vi "ELVIS III v1.1 Start AO Continuous.vi"(8 "error in (no error)":errorcluster, 9 "AO FIFO Sample Rate":dbl=1000.0 min=1000.0 max=1600000.0, 10 "Channel Info":T1, 11 "myRIO Ref In":T2) -> (0 "error out":errorcluster, 2 "Channel Info Out":T1, 3 "myRIO Ref Out":T2)   [LabVIEW 2021]
uses:
  <vilib>/myRIO/Common/Instrument Driver Framework/Utilities/typedefs/myRIO v1.0 Reference.ctl
  <vilib>/myRIO/Common/Instrument Driver Framework/Utilities/typedefs/Generic FPGA Reference.ctl
  <vilib>/myRIO/Common/Instrument Driver Framework/ELVIS III v1.0/AO Continuous/typedefs/AO Continuous Channel Info.ctl
  <vilib>/myRIO/Common/Instrument Driver Framework/ELVIS III v1.0/AO Block/typedefs/ELVIS III AO Block Channels FPGA Reference.ctl
  <vilib>/rvi/errors/niLvFpgaAdjustHostInterfaceError.vi
  <vilib>/rvi/interface/nirviReadWriteControl/nirviReadWriteControl.xnode
  NiFpgaLv.dll
  <vilib>/rvi/interface/Simulation/niFpgaSimulationCallBeginRW.vi
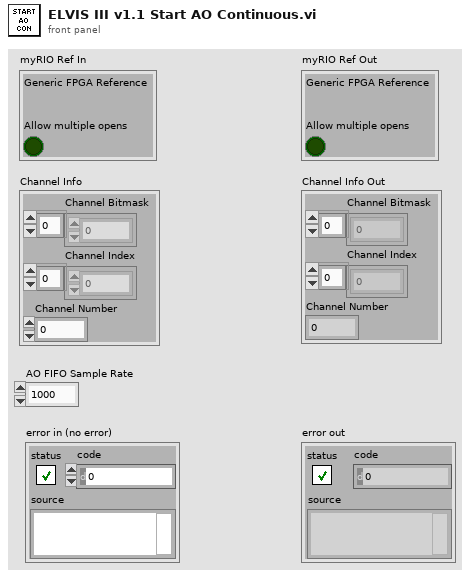
[diagram p1: front panel]
types:
  T1 = typedef "AO Continuous Channel Info.ctl" = cluster{"Channel Bitmask":u8[], "Channel Index":i32[], "Channel Number":u8}
  T2 = typedef "myRIO v1.0 Reference.ctl" = cluster{"Generic FPGA Reference":T3, "Allow multiple opens":bool}
  T3 = typedef "Generic FPGA Reference.ctl" = refnum<k20>
  T4 = typedef "ELVIS III AO Block Channels FPGA Reference.ctl" = refnum<k20>
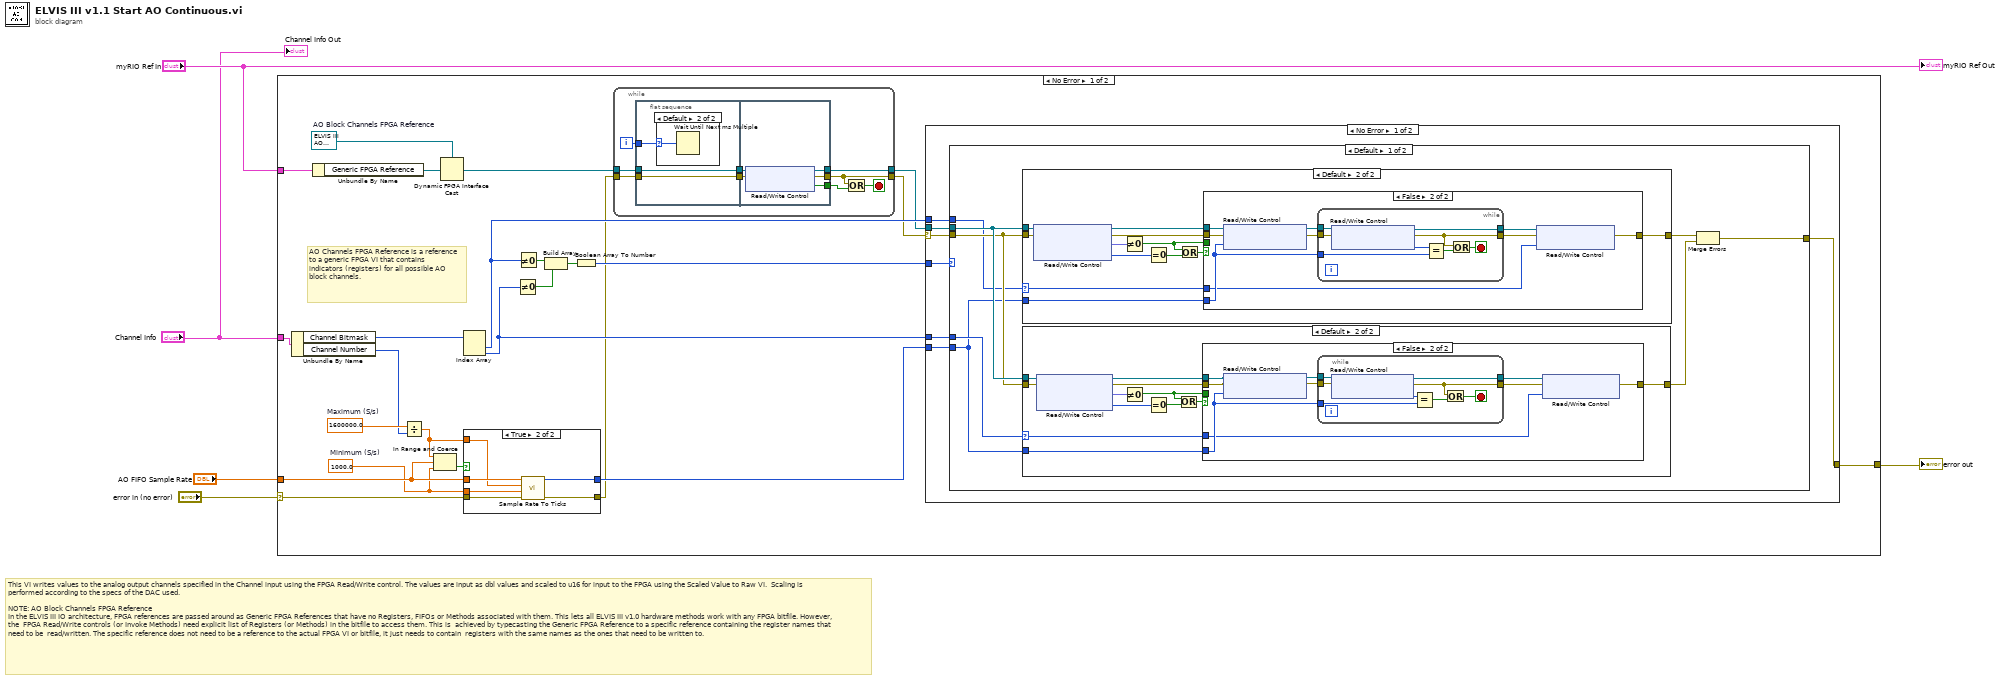
[diagram p0: block diagram]
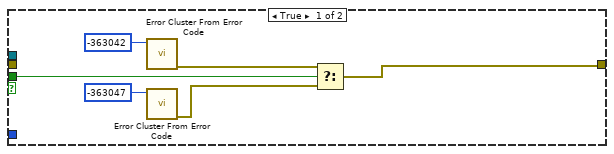
[diagram p3: hidden frame]
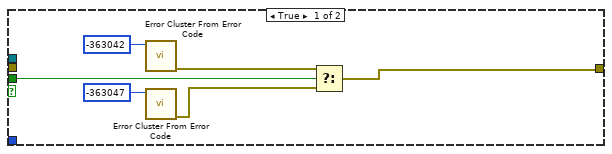
[diagram p5: hidden frame]
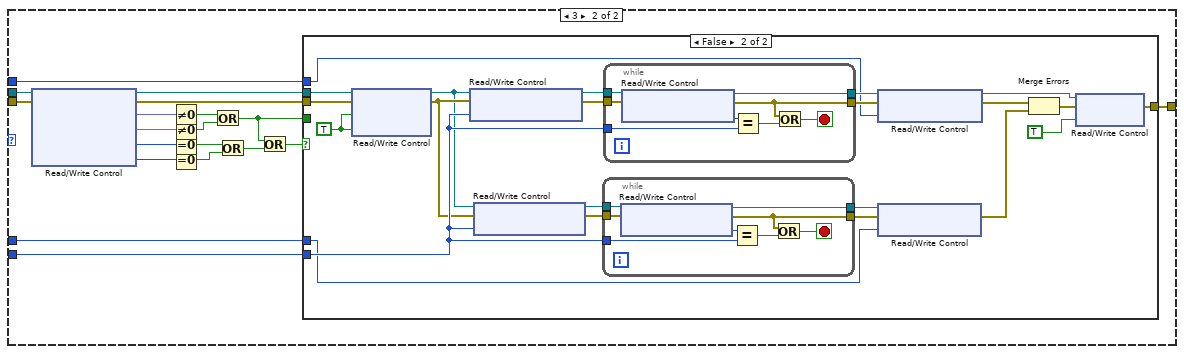
[diagram p6: hidden frame]
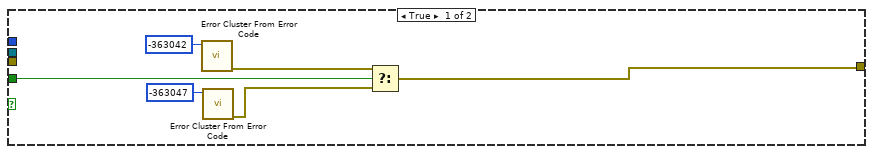
[diagram p7: hidden frame]
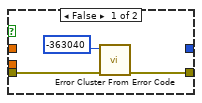
[diagram p10: hidden frame]
diagram:
  # "This VI writes values to the analog output channels specified in the Channel input using the FPGA Read/Write control. The values are input as dbl values and scaled to u16 for input to the FPGA using the Scaled Value to Raw VI.  Scaling is performed according to the specs of the DAC used.\n\nNOTE: AO Block Channels FPGA Reference\nIn the ELVIS III IO architecture, FPGA references are passed around as Generic FPGA References that have no Registers, FIFOs or Methods associated with them. This lets all ELVIS III v1.0 hardware methods work with any FPGA bitfile. However, the  FPGA Read/Write controls (or Invoke Methods) need explicit list of Registers (or Methods) in the bitfile to access them. This is  achieved by typecasting the Generic FPGA Reference to a specific reference containing the register names that need to be  read/written. The specific reference does not need to be a reference to the actual FPGA VI or bitfile, it just needs to contain  registers with the same names as the ones that need to be written to."
  n1 = case shown="No Error" "error in (no error)" {
    selector: "error in (no error)" -> [w13 w208]
    tunnel: [w14 w208] -> w5
    tunnel: "AO FIFO Sample Rate" -> [w26 _]
    tunnel: "myRIO Ref In" -> [w28 _]
    tunnel: "Channel Info" -> [w18 _]
    frame No Error {
      w24 = 1000.0  # Minimum (S/s)
      w12 = 1600000.0  # Maximum (S/s)
      w27 = T4 refnum  # AO Block Channels FPGA Reference
      # "AO Channels FPGA Reference is a reference to a generic FPGA VI that contains indicators (registers) for all possible AO block channels."
      n2 = Unbundle By Name(w18) -> ("Channel Bitmask"=w17:u8[], "Channel Number"=w11:u8)
      n3 = Unbundle By Name(w28) -> ("Generic FPGA Reference"=w29:T3)
      n4 = Divide(x=w12, y=w11) -> (x/y=w10:dbl)
      n5 = In Range and Coerce(upper limit=w10, x=w26, lower limit=w24) -> (In Range?=w25:bool)  [unwired: 1 out]
      n6 = Dynamic FPGA Interface Cast(Session In=w27, Type=w29) -> (Session Out=w9:T4)
      n7 = Index Array(array=w17) -> (element #1=w16:u8, element #2=w15:u8)  [unwired: 2 in]
      n8 = case shown="True" w25 {
        tunnel: [_ w207] -> w19
        tunnel: w13 -> [w200 w206]
        tunnel: [w199 w205] -> w8
        tunnel: w26 -> [_ w204]
        tunnel: w24 -> [_ w203]
        tunnel: w10 -> [_ w202]
        frame False {
          n9 = call <vilib>:"Error Cluster From Error Code.vi"("error in (no error)"=w200, "error code (0)"=-363040) -> ("error out"=w199:errorcluster)  [unwired: 7 in]
        }
        frame True {
          n10 = call <vilib>:"Sample Rate To Ticks.vi"("error in (no error)"=w206, "Minimum (S/s)"=w203, "Maximum (S/s)"=w202, "Sample Rate (S/s)"=w204) -> ("error out"=w205:errorcluster, "Count (tick/s)"=w207:u32)  [unwired: 5 in, 1 out]
        }
      }
      n11 = Not Equal To 0?(x=w15) -> (x != 0?=w21:bool)
      n12 = Not Equal To 0?(x=w16) -> (x != 0?=w22:bool)
      n13 = Build Array(w22, w21) -> (w23:bool[])
      n14 = Boolean Array To Number(Boolean array=w23) -> (number=w20:u32)
      n15 = while {
        tunnel: w9 -> [w189]
        tunnel: w8 -> [w188]
        tunnel: [w184] -> w6
        tunnel: [w187] -> w7
        i -> [w181]
        stop <- w182 stop-if-true
        n16 = flat-sequence {
          tunnel: w188 -> [w191]
          tunnel: w189 -> [w192]
          tunnel: [w192] -> w186
          tunnel: [w191] -> w185
          tunnel: w181 -> [w190]
          tunnel: [w196] -> w183
          tunnel: [w195] -> w184
          tunnel: [w194] -> w187
          tunnel: w186 -> [w198]
          tunnel: w185 -> [w197]
          frame #0 {
            n17 = case shown="Default" w190 {
              selector: w190 -> [_ w193]
              frame 0 {
              }
              frame Default {
                n18 = Wait Until Next ms Multiple(millisecond multiple=w193) -> ()  [unwired: 1 out]
              }
            }
          }
          frame #1 {
            n19 = xnode "Read/Write Control"("FPGA VI Reference In"=w198, "error in"=w197) -> ("FPGA VI Reference Out"=w194:T4, "error out"=w195:errorcluster, "DMA.SYS.RDY"=w196:bool)
          }
        }
        n20 = Or(x=w184, y=w183) -> (x .or. y?=w182:bool)
      }
      n21 = case shown="No Error" w6 {
        selector: w6 -> [w30 w180]
        tunnel: w20 -> [w36 _]
        tunnel: w19 -> [w35 _]
        tunnel: w16 -> [w34 _]
        tunnel: w15 -> [w33 _]
        tunnel: [w32 w180] -> w14
        tunnel: w7 -> [w31 _]
        frame No Error {
          n22 = case shown="Default" w36 {
            tunnel: w31 -> [w44 w129]
            tunnel: w30 -> [w43 w128]
            tunnel: w34 -> [w42 w132]
            tunnel: w35 -> [w40 w135]
            tunnel: w33 -> [w41 w134]
            tunnel: [w39 w133] -> w32
            frame Default {
              n23 = case shown="Default" w42 {
                selector: w42 -> [_ w93]
                tunnel: w44 -> [_ w90]
                tunnel: w43 -> [w81 w89]
                tunnel: w40 -> [_ w92]
                tunnel: [w81 w91] -> w38
                frame 0 {
                }
                frame Default {
                  n24 = xnode "Read/Write Control"("FPGA VI Reference In"=w90, "error in"=w89) -> ("FPGA VI Reference Out"=w87:T4, "error out"=w88:errorcluster, "AO.A.DMA_ENA"=w86:fxp<+,2,2>, "AO.A.ELE_NUM"=w83:u32)
                  n25 = Not Equal To 0?(x=w86) -> (x != 0?=w84:bool)
                  n26 = Equal To 0?(x=w83) -> (x = 0?=w82:bool)
                  n27 = Or(x=w84, y=w82) -> (x .or. y?=w85:bool)
                  n28 = case shown="False" w85 {
                    tunnel: w88 -> [_ w107]
                    tunnel: [w96 w101] -> w91
                    tunnel: w87 -> [_ w108]
                    tunnel: w93 -> [_ w100]
                    tunnel: w92 -> [_ w104]
                    tunnel: w84 -> [w98 _]
                    frame True {
                      n29 = call <vilib>:"Error Cluster From Error Code.vi"("error code (0)"=-363042) -> ("error out"=w97:errorcluster)  [unwired: 8 in]
                      n30 = call <vilib>:"Error Cluster From Error Code.vi"("error code (0)"=-363047) -> ("error out"=w94:errorcluster)  [unwired: 8 in]
                      n31 = Select(t=w97, s=w98, f=w94) -> (s? t:f=w96:errorcluster)
                    }
                    frame False {
                      n32 = xnode "Read/Write Control"("FPGA VI Reference In"=w108, "error in"=w107, "AO.A.DMA_CNTR"=w104) -> ("FPGA VI Reference Out"=w106:T4, "error out"=w105:errorcluster)
                      n33 = while {
                        tunnel: w106 -> [w116]
                        tunnel: [w115] -> w103
                        tunnel: [w111] -> w102
                        tunnel: w105 -> [w114]
                        tunnel: w104 -> [w112]
                        stop <- w110 stop-if-true
                        n34 = xnode "Read/Write Control"("FPGA VI Reference In"=w116, "error in"=w114) -> ("FPGA VI Reference Out"=w115:T4, "error out"=w111:errorcluster, "AO.A.DMA_CNTR"=w113:u32)
                        n35 = Equal?(x=w113, y=w112) -> (x = y?=w109:bool)
                        n36 = Or(x=w111, y=w109) -> (x .or. y?=w110:bool)
                      }
                      n37 = xnode "Read/Write Control"("FPGA VI Reference In"=w103, "error in"=w102, "AO.A.DMA_ENA"=w100) -> ("error out"=w101:errorcluster)  [unwired: 1 out]
                    }
                  }
                }
              }
              n38 = case shown="Default" w41 {
                selector: w41 -> [_ w57]
                tunnel: w44 -> [_ w54]
                tunnel: w43 -> [w45 w53]
                tunnel: w40 -> [_ w56]
                tunnel: [w45 w55] -> w37
                frame 0 {
                }
                frame Default {
                  n39 = xnode "Read/Write Control"("FPGA VI Reference In"=w54, "error in"=w53) -> ("FPGA VI Reference Out"=w51:T4, "error out"=w50:errorcluster, "AO.B.DMA_ENA"=w52:fxp<+,2,2>, "AO.B.ELE_NUM"=w47:u32)
                  n40 = Not Equal To 0?(x=w52) -> (x != 0?=w48:bool)
                  n41 = Equal To 0?(x=w47) -> (x = 0?=w46:bool)
                  n42 = Or(x=w48, y=w46) -> (x .or. y?=w49:bool)
                  n43 = case shown="False" w49 {
                    tunnel: w50 -> [_ w71]
                    tunnel: [w58 w64] -> w55
                    tunnel: w51 -> [_ w72]
                    tunnel: w57 -> [_ w67]
                    tunnel: w56 -> [_ w68]
                    tunnel: w48 -> [w62 _]
                    frame True {
                      n44 = call <vilib>:"Error Cluster From Error Code.vi"("error code (0)"=-363042) -> ("error out"=w61:errorcluster)  [unwired: 8 in]
                      n45 = call <vilib>:"Error Cluster From Error Code.vi"("error code (0)"=-363047) -> ("error out"=w59:errorcluster)  [unwired: 8 in]
                      n46 = Select(t=w61, s=w62, f=w59) -> (s? t:f=w58:errorcluster)
                    }
                    frame False {
                      n47 = xnode "Read/Write Control"("FPGA VI Reference In"=w72, "error in"=w71, "AO.B.DMA_CNTR"=w68) -> ("FPGA VI Reference Out"=w70:T4, "error out"=w69:errorcluster)
                      n48 = while {
                        tunnel: w70 -> [w80]
                        tunnel: [w79] -> w66
                        tunnel: [w74] -> w65
                        tunnel: w69 -> [w78]
                        tunnel: w68 -> [w76]
                        stop <- w73 stop-if-true
                        n49 = xnode "Read/Write Control"("FPGA VI Reference In"=w80, "error in"=w78) -> ("FPGA VI Reference Out"=w79:T4, "error out"=w74:errorcluster, "AO.B.DMA_CNTR"=w77:u32)
                        n50 = Equal?(x=w77, y=w76) -> (x = y?=w75:bool)
                        n51 = Or(x=w74, y=w75) -> (x .or. y?=w73:bool)
                      }
                      n52 = xnode "Read/Write Control"("FPGA VI Reference In"=w66, "error in"=w65, "AO.B.DMA_ENA"=w67) -> ("error out"=w64:errorcluster)  [unwired: 1 out]
                    }
                  }
                }
              }
              n53 = Merge Errors(w38, w37) -> (w39:errorcluster)
            }
            frame 3 {
              n54 = xnode "Read/Write Control"("FPGA VI Reference In"=w129, "error in"=w128) -> ("FPGA VI Reference Out"=w131:T4, "error out"=w130:errorcluster, "AO.A.DMA_ENA"=w127:fxp<+,2,2>, "AO.B.DMA_ENA"=w126:fxp<+,2,2>, "AO.A.ELE_NUM"=w120:u32, "AO.B.ELE_NUM"=w119:u32)
              n55 = Not Equal To 0?(x=w127) -> (x != 0?=w125:bool)
              n56 = Not Equal To 0?(x=w126) -> (x != 0?=w124:bool)
              n57 = Equal To 0?(x=w120) -> (x = 0?=w118:bool)
              n58 = Equal To 0?(x=w119) -> (x = 0?=w117:bool)
              n59 = Or(x=w125, y=w124) -> (x .or. y?=w121:bool)
              n60 = Or(x=w118, y=w117) -> (x .or. y?=w123:bool)
              n61 = Or(x=w121, y=w123) -> (x .or. y?=w122:bool)
              n62 = case shown="False" w122 {
                tunnel: w131 -> [_ w156]
                tunnel: w130 -> [_ w158]
                tunnel: w132 -> [_ w146]
                tunnel: w134 -> [_ w142]
                tunnel: w135 -> [_ w159]
                tunnel: [w137 w152] -> w133
                tunnel: w121 -> [w139 _]
                frame True {
                  n63 = call <vilib>:"Error Cluster From Error Code.vi"("error code (0)"=-363042) -> ("error out"=w141:errorcluster)  [unwired: 8 in]
                  n64 = call <vilib>:"Error Cluster From Error Code.vi"("error code (0)"=-363047) -> ("error out"=w138:errorcluster)  [unwired: 8 in]
                  n65 = Select(t=w141, s=w139, f=w138) -> (s? t:f=w137:errorcluster)
                }
                frame False {
                  w154 = TRUE ("AO.A.SYNC")
                  n66 = xnode "Read/Write Control"("FPGA VI Reference In"=w156, "error in"=w158, "AO.A.SYNC"=w154, "AO.B.SYNC"=w154) -> ("FPGA VI Reference Out"=w155:T4, "error out"=w157:errorcluster)
                  n67 = xnode "Read/Write Control"("FPGA VI Reference In"=w155, "error in"=w157, "AO.A.DMA_CNTR"=w159) -> ("FPGA VI Reference Out"=w163:T4, "error out"=w162:errorcluster)
                  n68 = xnode "Read/Write Control"("FPGA VI Reference In"=w155, "error in"=w157, "AO.B.DMA_CNTR"=w159) -> ("FPGA VI Reference Out"=w161:T4, "error out"=w160:errorcluster)
                  n69 = while {
                    tunnel: w161 -> [w171]
                    tunnel: [w170] -> w145
                    tunnel: [w165] -> w144
                    tunnel: w160 -> [w169]
                    tunnel: w159 -> [w167]
                    stop <- w164 stop-if-true
                    n70 = xnode "Read/Write Control"("FPGA VI Reference In"=w171, "error in"=w169) -> ("FPGA VI Reference Out"=w170:T4, "error out"=w165:errorcluster, "AO.B.DMA_CNTR"=w168:u32)
                    n71 = Equal?(x=w168, y=w167) -> (x = y?=w166:bool)
                    n72 = Or(x=w165, y=w166) -> (x .or. y?=w164:bool)
                  }
                  n73 = while {
                    tunnel: w163 -> [w179]
                    tunnel: [w174] -> w150
                    tunnel: w162 -> [w178]
                    tunnel: w159 -> [w176]
                    tunnel: [w172] -> w149
                    stop <- w173 stop-if-true
                    n74 = xnode "Read/Write Control"("FPGA VI Reference In"=w179, "error in"=w178) -> ("FPGA VI Reference Out"=w172:T4, "error out"=w174:errorcluster, "AO.A.DMA_CNTR"=w177:u32)
                    n75 = Equal?(x=w177, y=w176) -> (x = y?=w175:bool)
                    n76 = Or(x=w174, y=w175) -> (x .or. y?=w173:bool)
                  }
                  n77 = xnode "Read/Write Control"("FPGA VI Reference In"=w149, "error in"=w150, "AO.A.DMA_ENA"=w146) -> ("FPGA VI Reference Out"=w148:T4, "error out"=w147:errorcluster)
                  n78 = xnode "Read/Write Control"("FPGA VI Reference In"=w145, "error in"=w144, "AO.B.DMA_ENA"=w142) -> ("error out"=w143:errorcluster)  [unwired: 1 out]
                  n79 = Merge Errors(w147, w143) -> (w153:errorcluster)
                  n80 = xnode "Read/Write Control"("FPGA VI Reference In"=w148, "error in"=w153, "AO.SYNC"=TRUE ("AO.A.SYNC")) -> ("error out"=w152:errorcluster)  [unwired: 1 out]
                }
              }
            }
          }
        }
        frame Error {
        }
      }
    }
    frame Error {
      # "There is an incoming error so there is nothing to do."
    }
  }
  "error out" <- w5
  "myRIO Ref Out" <- "myRIO Ref In"
  "Channel Info Out" <- "Channel Info"
